vi "testWaitTimerCancel.vi"(8 "error in (no error)":errorcluster, 11 "testStateMachineUtilities in":refnum<class "testStateMachineUtilities.lvclass">) -> (0 "error out":errorcluster, 3 "testStateMachineUtilities out":refnum<class "testStateMachineUtilities.lvclass">)   [LabVIEW 2013, in "testStateMachineUtilities.lvclass"]
uses:
  testStateMachineUtilities.lvclass
  <vilib>/Utility/error.llb/Error Cluster From Error Code.vi
panel:
  out "Array 3":string[](array[string])
  out "Array 2":string[](array[string])
  out "Array":string[](array[string])
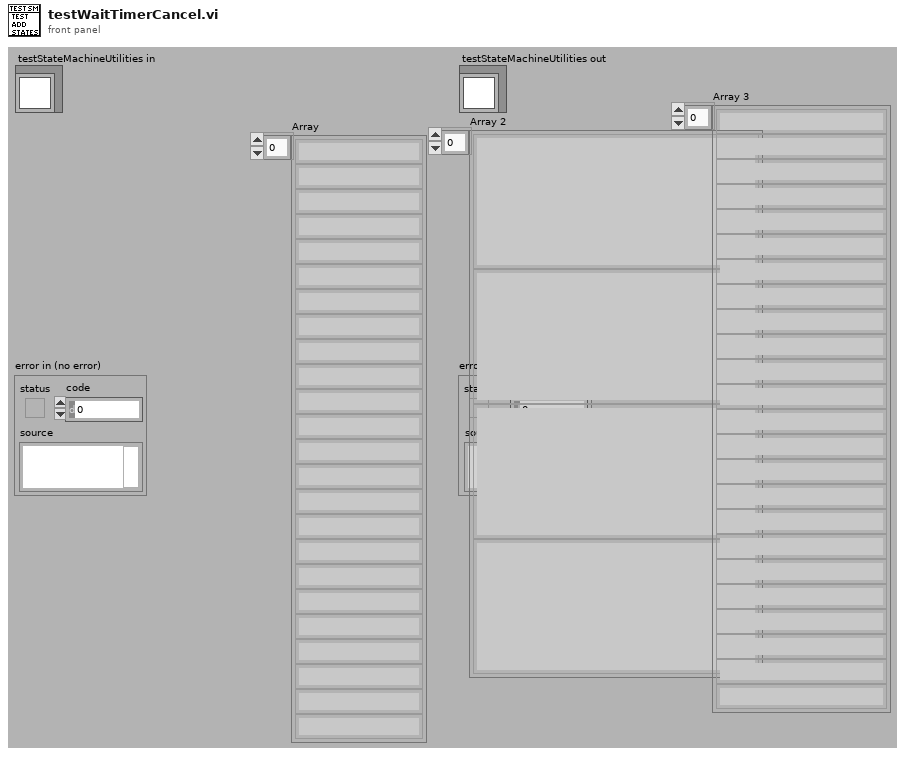
[diagram p1: front panel]
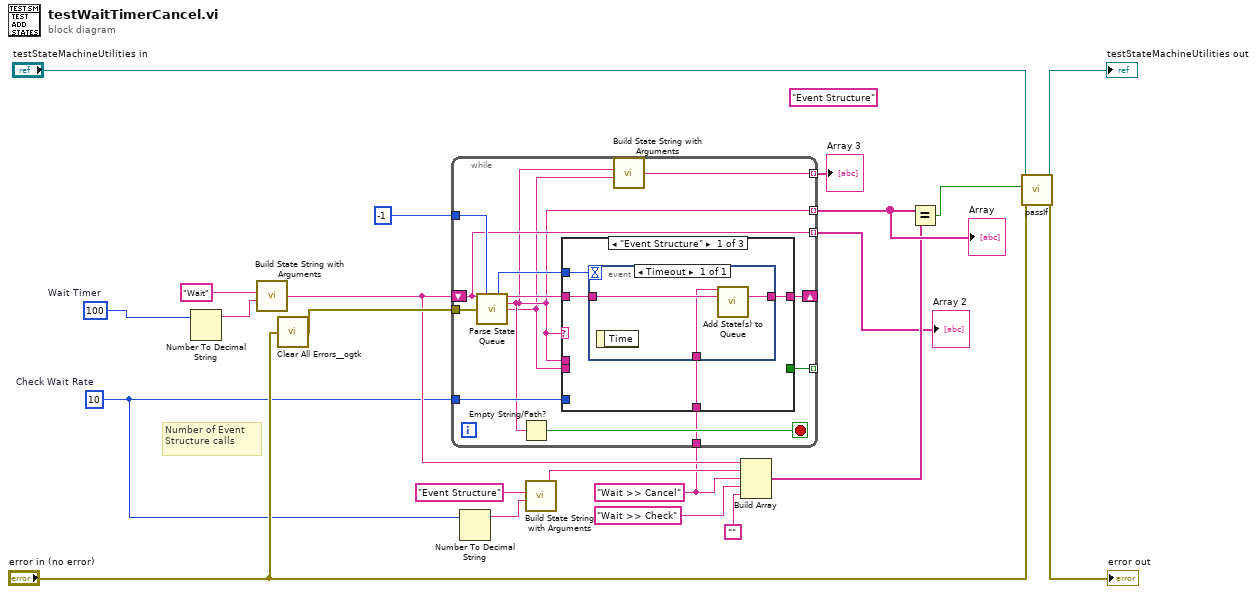
[diagram p0: block diagram]
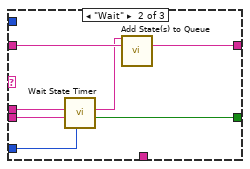
[diagram p2: hidden frame]
diagram:
  w1 = "Wait >> Cancel" ("State Queue")
  (unwired) "Event Structure" ("State Queue")
  w9 = 100  # Wait Timer
  w5 = 10  # Check Wait Rate
  # "Number of Event Structure calls"
  n1 = Number To Decimal String(number=w9) -> (decimal integer string=w14:string)  [unwired: 1 in]
  n2 = call "Build State String with Arguments.vi"("Arguments (\"\")"=w14, "State"="Wait" ("State Queue")) -> ("State with Arguments"=w8:string)  [unwired: 4 in]
  n3 = call <userlib>:"Clear All Errors__ogtk.vi"("Error In"="error in (no error)") -> ("Error Out"=w18:errorcluster)  [unwired: 3 in]
  n4 = while {
    tunnel: w18 -> [w35]
    shift-right: [w30] -> _
    shift-left: w8 -> [w27]
    tunnel: -1 ("Timeout") -> [w34]
    tunnel: [w26] -> w13 mode=indexing
    tunnel: [w32] -> _ mode=indexing
    tunnel: w5 -> [w28]
    tunnel: [w27] -> w11 mode=indexing
    tunnel: [w24] -> w10 mode=indexing
    tunnel: w1 -> [w23]
    stop <- w33 stop-if-true
    n5 = call "Parse State Queue.vi"("State Queue"=w27, "Timeout"=w34, "Error In (no error)"=w35) -> ("Timeout out"=w29:i32, "Remaining States"=w31:string, "Current State"=w26:string, "Arguments"=w25:string)  [unwired: 9 in]
    n6 = Empty String/Path?(string/path=w26) -> (empty?=w33:bool)
    n7 = case shown="\"Event Structure\"" w26 {
      tunnel: w26 -> [_ w49 _]
      tunnel: w25 -> [_ w48 _]
      tunnel: [_ w47 _] -> w32
      tunnel: w31 -> [w38 w46 w50]
      tunnel: [w37 w45 w50] -> w30
      tunnel: w28 -> [_ w43 _]
      tunnel: w29 -> [w39 _ _]
      tunnel: w23 -> [w36 _ _]
      frame "Event Structure" {
        n8 = event shown="[0] Timeout" {
          selector: _ -> [_]
          dyn-events: _ -> [_]
          timeout: w39 -> [_]
          tunnel: w38 -> [w41]
          tunnel: [w42] -> w37
          tunnel: w36 -> [w40]
          event Timeout {
            n9 = event-data() -> ()  [unwired: 1 in, 1 out]
            n10 = call "Add State(s) to Queue.vi"("State(s) in Front (\"\")"=w40, "State(s) in (\"\")"=w41) -> ("States Out"=w42:string)  [unwired: 13 in]
          }
        }
      }
      frame "Wait" {
        n11 = call "Wait State Timer.vi"("Check Wait Rate"=w43, "Wait Time (Decimal String)"=w48, "Current State"=w49) -> ("Wait Timer Elapsed"=w47:bool, "States to Enqueue"=w44:string)  [unwired: 5 in, 2 out]
        n12 = call "Add State(s) to Queue.vi"("State(s) in Front (\"\")"=w44, "State(s) in (\"\")"=w46) -> ("States Out"=w45:string)  [unwired: 13 in]
      }
      frame Default {
      }
    }
    n13 = call "Build State String with Arguments.vi"("Arguments (\"\")"=w25, "State"=w26) -> ("State with Arguments"=w24:string)  [unwired: 4 in]
  }
  "Array" <- w13
  "Array 2" <- w11
  "Array 3" <- w10
  n14 = Number To Decimal String(number=w5) -> (decimal integer string=w7:string)  [unwired: 1 in]
  n15 = call "Build State String with Arguments.vi"("Arguments (\"\")"=w7, "State"="Event Structure" ("State Queue")) -> ("State with Arguments"=w4:string)  [unwired: 4 in]
  n16 = Build Array(w8, w4, w1, "Wait >> Check" ("State Queue"), "") -> (w12:string[])
  n17 = Equal?(x=w13, y=w12) -> (x = y?=w16:bool)
  n18 = call-dynamic "passIf.vi"("error in (no error)"="error in (no error)", "pass"=w16, "TestCase in"="testStateMachineUtilities in") -> ("error out"=→"error out":errorcluster, "TestCase out"=→"testStateMachineUtilities out":refnum<class "testStateMachineUtilities.lvclass">)  [unwired: 7 in]
